vi "Draw Text For Demo.vi"(9 "color":u32, 10 "text":string, 11 "picture in":picture) -> (3 "picture out":picture)   [LabVIEW 2023]
doc: "This VI draws text into a picture at a random vertical position useful for the example."
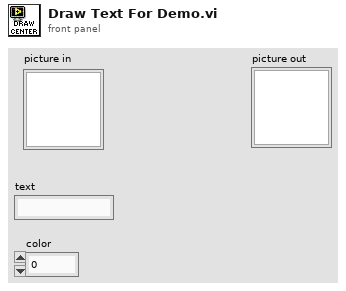
[diagram p1: front panel]
types:
  T1 = cluster{"horizontal":enum16{"left", "center", "right"}, "vertical":enum16{"top", "center", "bottom"}}
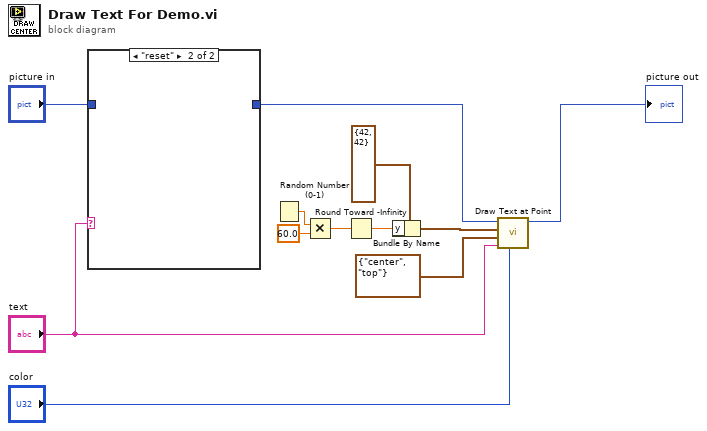
[diagram p0: block diagram]
diagram:
  n1 = case shown="\"reset\"" "text" {
    tunnel: [w13 _] -> w2
    tunnel: "picture in" -> [w13 _]
    frame Default {
    }
    frame "reset" {
    }
  }
  n2 = Random Number (0-1)() -> (number: 0 to 1=w7:dbl)
  n3 = Multiply(x=w7, y=60.0) -> (x*y=w5:dbl)
  n4 = Round Toward -Infinity(1:w5) -> (0:w4:dbl)
  n5 = Bundle By Name(cluster=cluster{"x":i16, "y":i16} {"x"=42, "y"=42} ("origin"), "y"=w4) -> (w8:cluster{"x":i16, "y":i16})
  n6 = call <vilib>:"Draw Text at Point.vi"("text color(black)"="color", "text"="text", "alignment(left, top)"=T1 {"horizontal"=enum."center", "vertical"=enum."top"}, "origin"=w8, "picture"=w2) -> ("new picture"=→"picture out":picture)  [unwired: 5 in, 1 out]
